vi "PositionBased1DProfile.vi"(9 "MaxAccel":dbl, 10 "MaxVel":dbl, 11 "Distance":dbl) -> (3 "Profile":cluster{"Distances":dbl[], "Vels":dbl[]})   [LabVIEW 2017]
panel:
  out "XY Graph":cluster{dbl[], dbl[]}(graph)
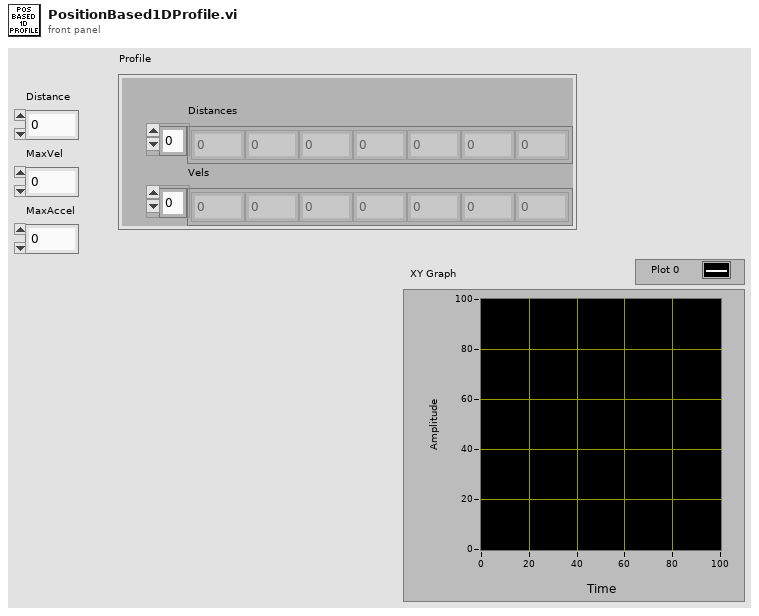
[diagram p1: front panel]
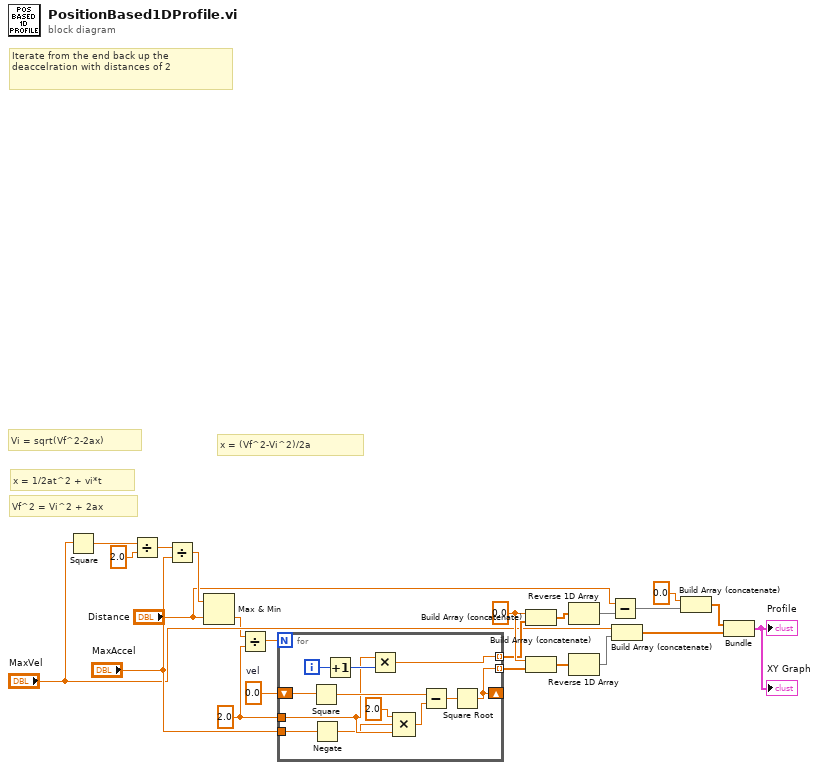
[diagram p0: block diagram]
diagram:
  w11 = 0.0 ("y")
  w19 = 0.0  # vel
  w20 = 2.0 ("y")
  # "Vi = sqrt(Vf^2-2ax)"
  # "Iterate from the end back up the\ndeaccelration with distances of 2"
  # "x = (Vf^2-Vi^2)/2a"
  # "Vf^2 = Vi^2 + 2ax"
  # "x = 1/2at^2 + vi*t"
  n1 = Square(x="MaxVel") -> (x^2=w21:dbl)
  n2 = Divide(x=w21, y=2.0) -> (x/y=w22:dbl)
  n3 = Divide(x=w22, y="MaxAccel") -> (x/y=w13:dbl)
  n4 = Max & Min(x=w13, y="Distance") -> (min(x,y)=w3:dbl)  [unwired: 1 out]
  n5 = Divide(x=w3, y=w20) -> (x/y=w12:dbl)
  n6 = for {
    N: w12 -> [_]
    tunnel: w20 -> [w30]
    shift-right: [w27] -> _
    shift-left: w19 -> [w33]
    tunnel: "MaxAccel" -> [w26]
    tunnel: [w27] -> w10 mode=indexing
    tunnel: [w24] -> w9 mode=indexing
    i -> [w35]
    n7 = Square(x=w33) -> (x^2=w32:dbl)
    n8 = Negate(x=w26) -> (-x=w25:dbl)
    n9 = Increment(x=w35) -> (x+1=w34:i32)
    n10 = Multiply(x=w30, y=w34) -> (x*y=w24:dbl)
    n11 = Compound Arithmetic op=MULTIPLY(2.0 ("value"), w25, w30) -> (w29:dbl)
    n12 = Subtract(x=w32, y=w29) -> (x-y=w28:dbl)
    n13 = Square Root(x=w28) -> (sqrt(x)=w27:dbl)
  }
  n14 = Build Array (concatenate)(w11, w9) -> (w8:dbl[])
  n15 = Build Array (concatenate)(w11, w10) -> (w17:dbl[])
  n16 = Reverse 1D Array(array=w8) -> (reversed array=w4:dbl[])
  n17 = Reverse 1D Array(array=w17) -> (reversed array=w5:dbl[])
  n18 = Subtract(x="Distance", y=w4) -> (x-y=w2:dbl[])
  n19 = Build Array (concatenate)("MaxVel", w5) -> (w15:dbl[])
  n20 = Build Array (concatenate)(0.0 ("y"), w2) -> (w16:dbl[])
  n21 = Bundle(w16, w15) -> (→"Profile" →"XY Graph":cluster{dbl[], dbl[]})  [unwired: 1 in]
